vi "rad_Get Image Save Location.vi"(5 "Host Name":string, 7 "IP Address":string, 8 "error in (no error)":errorcluster, 10 "Starting Path":path=path "C:/dev/Architectures/Reference Designs/Application Deployment and Replication/Application Deployment Utility/trunk/source/Application Images", 11 "AppImage Properties":T1) -> (0 "error out":errorcluster, 1 "exists":bool, 2 "Application Image Path":path, 3 "AppImage Properties":T1, 4 "Cancelled":bool, 6 "Back":bool)   [LabVIEW 2016]
uses:
  TypeDefs/rad_Application Image Properties.ctl
  TypeDefs/rad_FPGA Properties.ctl
  TypeDefs/rad_FPGA Flash Properties.ctl
  Util/FP Control/FP Control Functions.ctl
panel:
  in  "Back":bool
  in  "Browse":bool
  in  "Cancel Button":bool
  in  "OK Button":bool
  # "Choose Image Storage Directory"
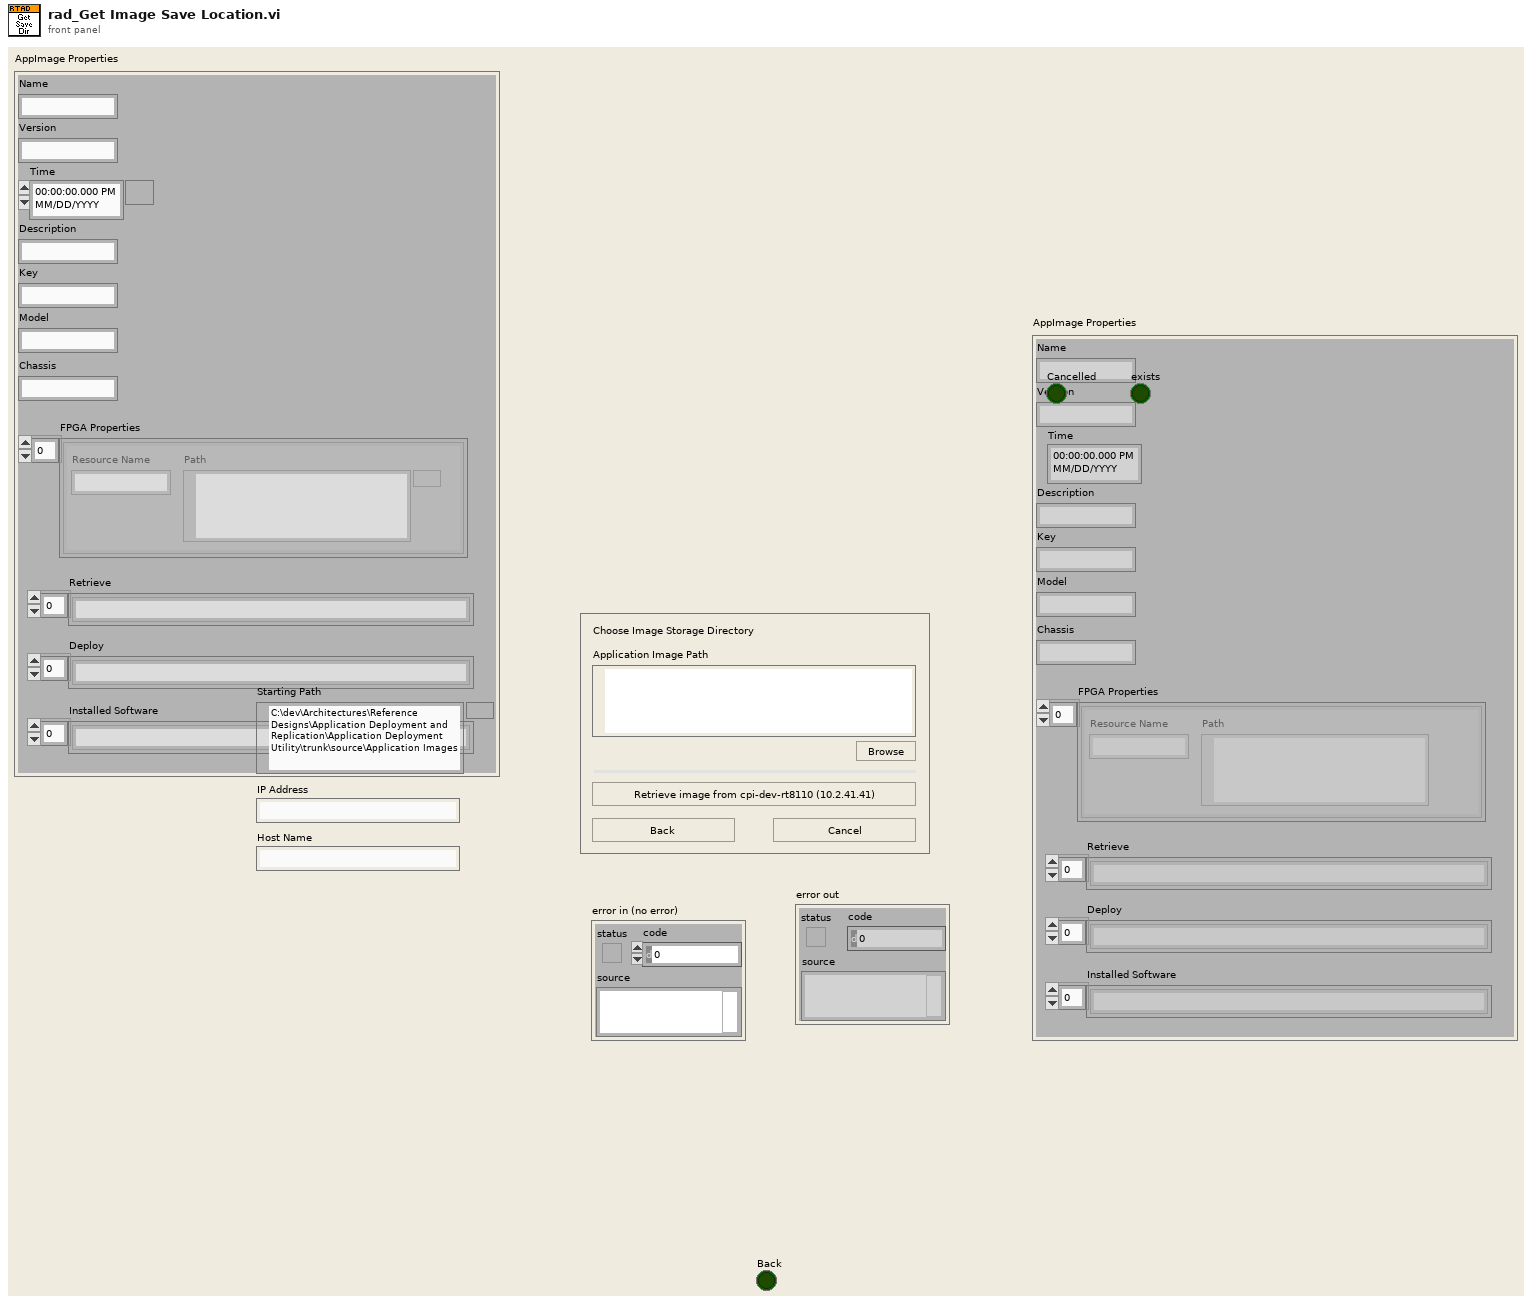
[diagram p1: front panel]
types:
  T1 = typedef "rad_Application Image Properties.ctl" = cluster{"Name":string, "Version":string, "Time":timestamp, "Description":string, "Key":string, "Chassis":string, "FPGA Properties":T2, "Model":string, "Retrieve":string[], "Deploy":string[], "Installed Software":string[]}
  T2 = typedef "rad_FPGA Properties.ctl" = T3[]
  T3 = typedef "rad_FPGA Flash Properties.ctl" = cluster{"Resource Name":string, "Path":path}
  T4 = typedef "FP Control Functions.ctl" = enum16{"Open", "Close", "Bring To Front", "Center"}
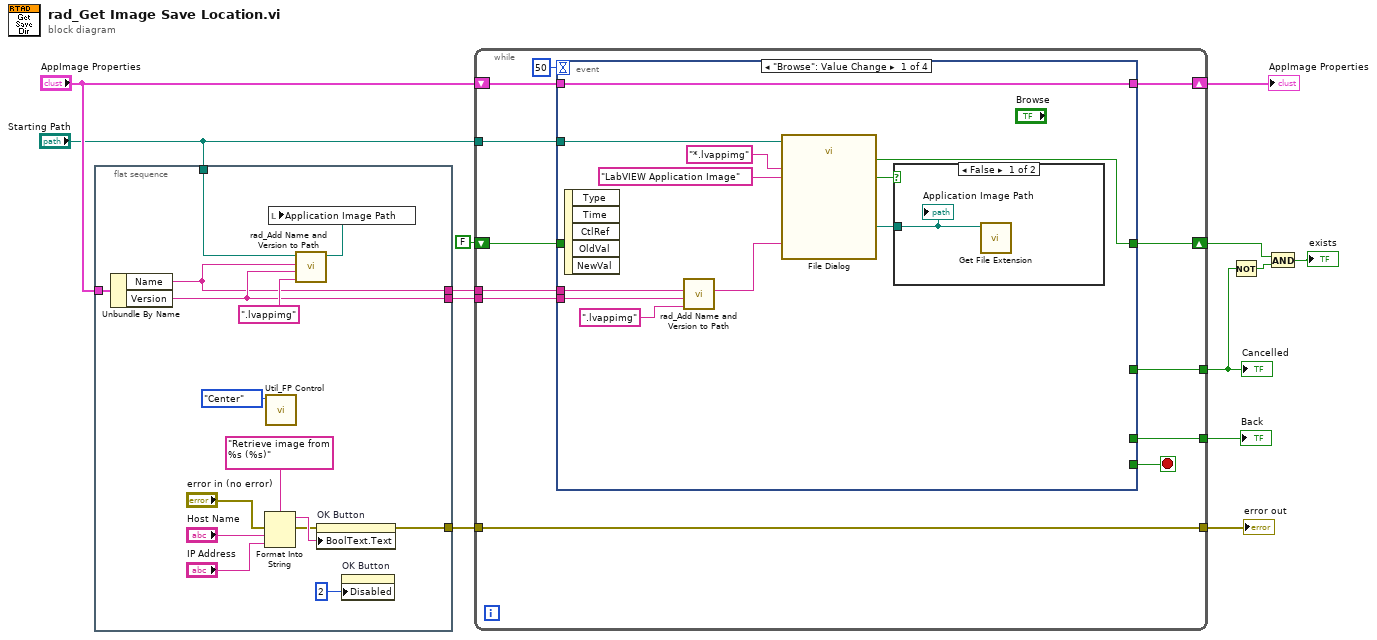
[diagram p0: block diagram]
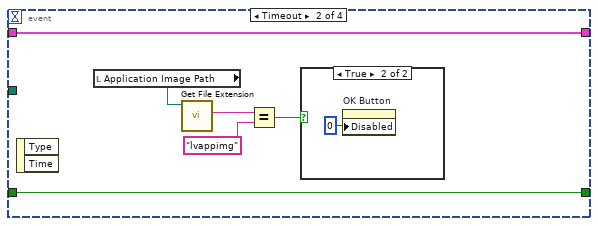
[diagram p3: hidden frame]
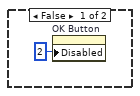
[diagram p4: hidden frame]
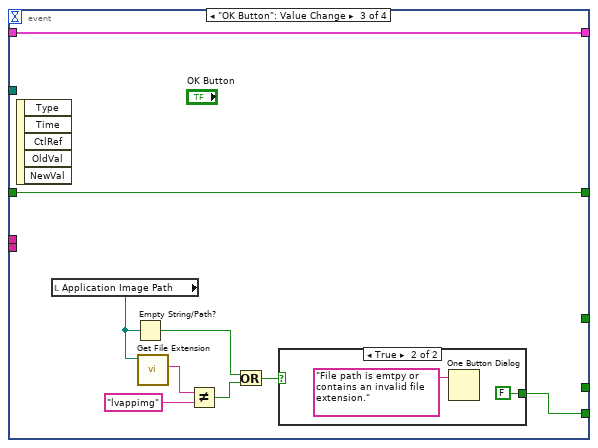
[diagram p5: hidden frame]
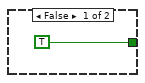
[diagram p6: hidden frame]
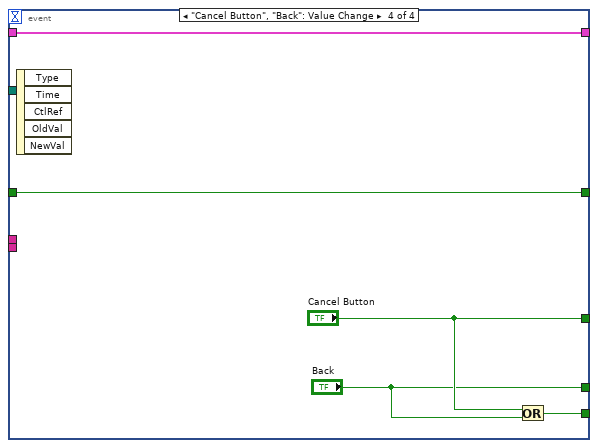
[diagram p7: hidden frame]
diagram:
  n1 = flat-sequence {
    tunnel: [w28] -> w13
    tunnel: "AppImage Properties" -> [w21]
    tunnel: "Starting Path" -> [w19]
    tunnel: [w15] -> w2
    tunnel: [w14] -> w3
    frame #0 {
      n2 = Unbundle By Name(w21) -> ("Name"=w14:string, "Version"=w15:string)
      n3 = Format Into String(format string="Retrieve image from %s (%s)", error in="error in (no error)", "Host Name", "IP Address") -> (resulting string=w24:string, error out=w22:errorcluster)  [unwired: 1 in]
      n4 = call "Util_FP Control.vi"("Function"=FP_Control_Functions."Center") -> ()  [unwired: 1 in, 10 out]
      n5 = call "rad_Add Name and Version to Path.vi"("File Extension"=".lvappimg", "Version"=w15, "Name"=w14, "Starting Path"=w19) -> ("New Path"=w18:path)  [unwired: 6 in, 1 out]
      n6 = local write "Application Image Path"(w18) -> ()
      n7 = property on="OK Button" class="Bool"(error in=w22, "BoolText.Text"=w24) -> (error out=w28:errorcluster)  [unwired: 1 in, 1 out]
      n8 = property on="OK Button" class="Bool"("Disabled"=2) -> ()  [unwired: 2 in, 2 out]
    }
  }
  n9 = while {
    tunnel: [w40] -> w12
    tunnel: w13 -> [w40]
    tunnel: "Starting Path" -> [w39]
    tunnel: [w37] -> w6
    shift-right: [w35] -> w4
    shift-left: "AppImage Properties" -> [w36]
    shift-right: [w34] -> w8
    shift-left: FALSE ("exists") -> [w33]
    tunnel: w3 -> [w31]
    tunnel: w2 -> [w30]
    tunnel: [w29] -> w1
    stop <- w38 stop-if-true
    n10 = event shown="[0] \"Browse\": Value Change" {
      selector: _ -> [_ _ _ _]
      dyn-events: _ -> [_ _ _ _]
      timeout: 50 -> [_ _ _ _]
      tunnel: w39 -> [w44 _ _ _]
      tunnel: [_ _ w69 w74] -> w38
      tunnel: [_ _ _ "Cancel Button"] -> w37
      tunnel: w36 -> [w47 w58 w68 w77]
      tunnel: [w47 w58 w68 w77] -> w35
      tunnel: [w46 w54 w67 w76] -> w34
      tunnel: w33 -> [_ w54 w67 w76]
      tunnel: w31 -> [w42 _ _ _]
      tunnel: w30 -> [w41 _ _ _]
      tunnel: [_ _ _ "Back"] -> w29
      event "Browse": Value Change {
        n11 = event-data() -> ()  [unwired: 1 in, 5 out]
        n12 = call "rad_Add Name and Version to Path.vi"("File Extension"=".lvappimg" ("pattern (all files)"), "Version"=w41, "Name"=w42) -> ("filename without extension"=w45:string)  [unwired: 7 in, 1 out]
        n13 = call "File Dialog"("start path"=w44, "default name"=w45, "pattern (all files)"="*.lvappimg", "pattern label"="LabVIEW Application Image") -> ("selected path"=w49:path, "exists"=w46:bool, "cancelled"=w50:bool)  [unwired: 3 in, 6 out]
        n14 = case shown="False" w50 {
          tunnel: w49 -> [w52 _]
          frame False {
            n15 = call <vilib>:"Get File Extension.vi"("file"=w52) -> ()  [unwired: 6 in, 5 out]
            "Application Image Path" <- w52
          }
          frame True {
          }
        }
      }
      event Timeout {
        n16 = event-data() -> ()  [unwired: 1 in, 2 out]
        n17 = local read "Application Image Path"() -> (w57:path)
        n18 = call <vilib>:"Get File Extension.vi"("file"=w57) -> ("lowercase file extension"=w56:string)  [unwired: 6 in, 4 out]
        n19 = Equal?(x=w56, y="lvappimg") -> (x = y?=w53:bool)
        n20 = case shown="True" w53 {
          frame False {
            n21 = property on="OK Button" class="Bool"("Disabled"=u8 2) -> ()  [unwired: 2 in, 2 out]
          }
          frame True {
            n22 = property on="OK Button" class="Bool"("Disabled"=u8 0) -> ()  [unwired: 2 in, 2 out]
          }
        }
      }
      event "OK Button": Value Change {
        n23 = event-data() -> ()  [unwired: 1 in, 5 out]
        n24 = local read "Application Image Path"() -> (w66:path)
        n25 = Empty String/Path?(string/path=w66) -> (empty?=w65:bool)
        n26 = call <vilib>:"Get File Extension.vi"("file"=w66) -> ("lowercase file extension"=w63:string)  [unwired: 6 in, 4 out]
        n27 = Not Equal?(x=w63, y="lvappimg" ("pattern (all files)")) -> (x != y?=w62:bool)
        n28 = Or(x=w65, y=w62) -> (x .or. y?=w61:bool)
        n29 = case shown="True" w61 {
          tunnel: [TRUE FALSE] -> w69
          frame False {
          }
          frame True {
            n30 = One Button Dialog(message="File path is emtpy or contains an invalid file extension.") -> ()  [unwired: 1 in, 1 out]
          }
        }
      }
      event "Cancel Button", "Back": Value Change {
        n31 = event-data() -> ()  [unwired: 1 in, 5 out]
        n32 = Or(x="Cancel Button", y="Back") -> (x .or. y?=w74:bool)
      }
    }
  }
  "Cancelled" <- w6
  "error out" <- w12
  "AppImage Properties" <- w4
  "Back" <- w1
  n33 = Not(x=w6) -> (.not. x?=w9:bool)
  n34 = And(x=w8, y=w9) -> (x .and. y?=→"exists":bool)
